vi "Select Best Address.vi"(8 "error in (no error)":errorcluster, 11 "addresses":refnum<class "Generic Network Address.lvclass">[](array[class])) -> (0 "error out":errorcluster, 2 "found?":bool, 3 "address":refnum<class "Generic Network Address.lvclass">)   [LabVIEW 2020, in "NI_WFCN.lvlib" / "Generic Network Address.lvclass"]
doc: "Given possibly more than one functionally equivalent address (e.g. the same host across different protocols), select the \"best\" one."
uses:
  <vilib>/net/WFCN/Addressing/Generic Network Address/Generic Network Address.lvclass
  <vilib>/net/WFCN/Addressing/IPv4 Network Address/IPv4 Network Address.lvclass
  e:/builds/penguin/labview/branches/2020/dev/dist/vi.lib/net/WFCN/Addressing/Generic Network Address/Generic Network Address.lvclass
  <vilib>/net/WFCN/Addressing/Hostname Network Address/Hostname Network Address.lvclass
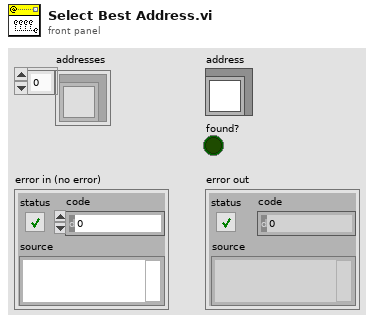
[diagram p1: front panel]
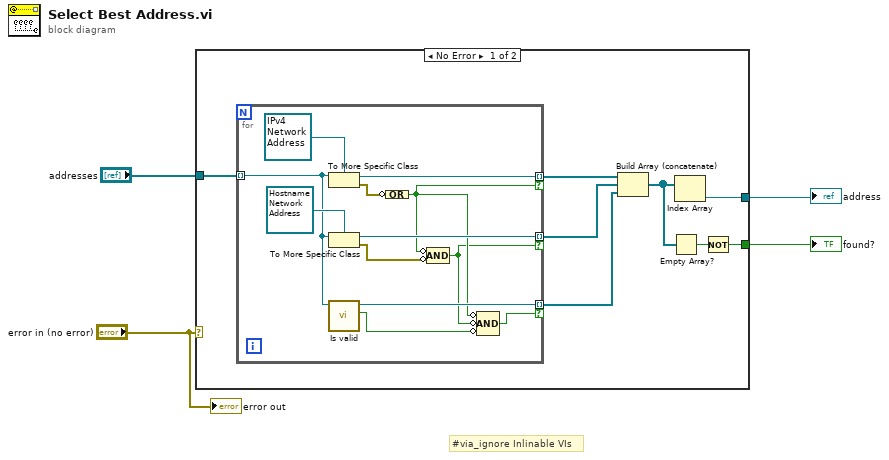
[diagram p0: block diagram]
diagram:
  # "#via_ignore Inlinable VIs"
  n1 = case shown="No Error" "error in (no error)" {
    tunnel: "addresses" -> [w12 _]
    tunnel: [w8 _] -> w3
    tunnel: [w5 _] -> w2
    frame No Error {
      n2 = for {
        tunnel: w12 -> [w20] mode=indexing
        tunnel: [w23] -> w11 mode=indexing if=w18
        tunnel: [w21] -> w10 mode=indexing if=w17
        tunnel: [w19] -> w9 mode=indexing if=w15
        n3 = To More Specific Class(target class=refnum<class "IPv4 Network Address.lvclass"> refnum ("WFCN.lvlib:IPv4 Network Address.lvclass"), reference=w20) -> (specific class reference=w23:refnum<class "IPv4 Network Address.lvclass">, error out=w14:errorcluster)  [unwired: 1 in]
        n4 = To More Specific Class(target class=refnum<class "Hostname Network Address.lvclass"> refnum ("WFCN.lvlib:Hostname Network Address.lvclass"), reference=w20) -> (specific class reference=w21:refnum<class "Hostname Network Address.lvclass">, error out=w13:errorcluster)  [unwired: 1 in]
        n5 = call-dynamic "Is valid.vi"("address"=w20) -> ("valid?"=w16:bool, "address out"=w19:refnum<class "Generic Network Address.lvclass">)  [unwired: 9 in]
        n6 = Compound Arithmetic op=OR(invert w14) -> (w18:bool)
        n7 = Compound Arithmetic op=AND(invert w18, invert w13) -> (w17:bool)
        n8 = Compound Arithmetic op=AND(invert w18, invert w17, invert w16) -> (w15:bool)
      }
      n9 = Build Array (concatenate)(w11, w10, w9) -> (w7:refnum<class "Generic Network Address.lvclass">[])
      n10 = Empty Array?(array=w7) -> (empty?=w6:bool)
      n11 = Index Array(array=w7) -> (element=w8:refnum<class "Generic Network Address.lvclass">)  [unwired: 1 in]
      n12 = Not(x=w6) -> (.not. x?=w5:bool)
    }
    frame Error {
    }
  }
  "address" <- w3
  "found?" <- w2
  "error out" <- "error in (no error)"
